vi "readSettingsFile.vi"(8 "error in (no error)":errorcluster, 10 "file (use dialog)":path, 11 "Controller in":refnum<class "Controller.lvclass">) -> (0 "error out":errorcluster, 3 "Controller out":refnum<class "Controller.lvclass">)   [LabVIEW 2019, in "Controller.lvclass"]
uses:
  Controller.lvclass
  Controller.lvclass/Controller.ctl
  Axis/Axis.lvclass
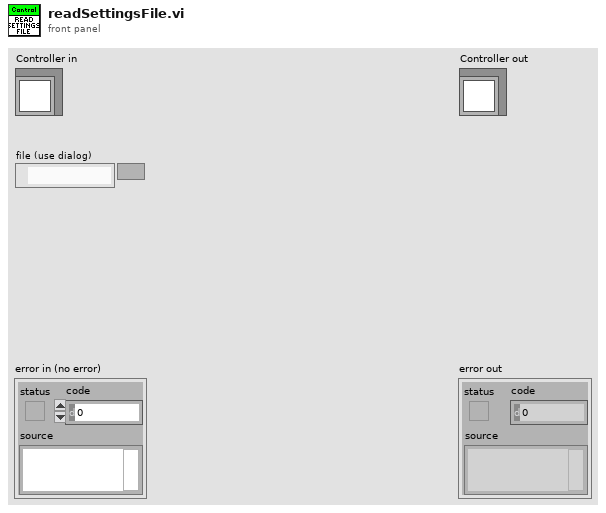
[diagram p1: front panel]
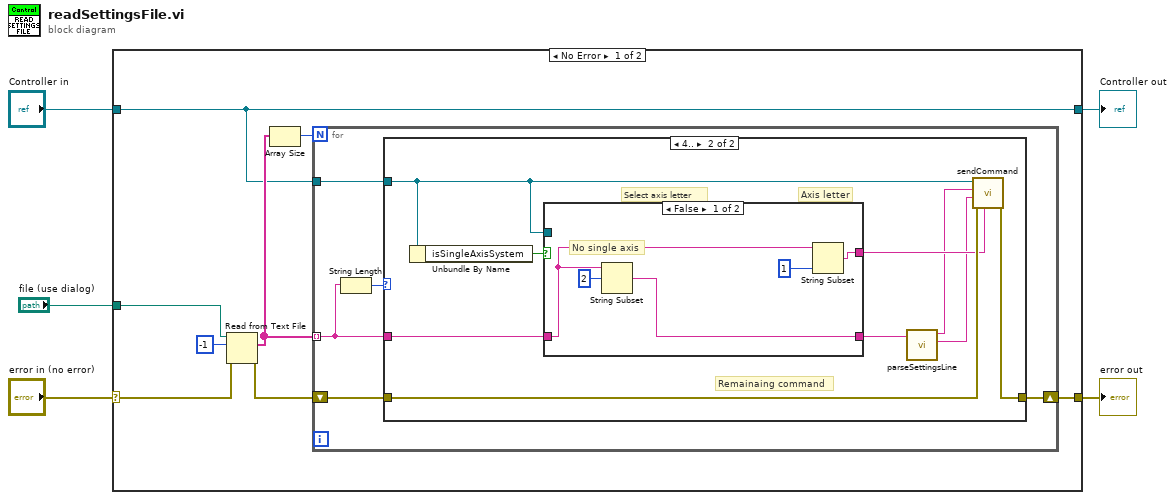
[diagram p0: block diagram]
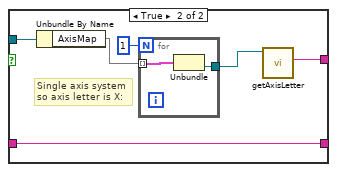
[diagram p3: hidden frame]
diagram:
  n1 = case shown="No Error" "error in (no error)" {
    selector: "error in (no error)" -> [w8 w43]
    tunnel: [w9 w43] -> w4
    tunnel: [w7 w42] -> w2
    tunnel: "Controller in" -> [w7 w42]
    tunnel: "file (use dialog)" -> [w6 _]
    frame No Error {
      n2 = Read from Text File(file (use dialog)=w6, count=-1, error in=w8) -> (text=w11:string[], error out=w10:errorcluster)  [unwired: 1 in, 2 out]
      n3 = Array Size(array=w11) -> (size(s)=w12:i32)
      n4 = for {
        N: w12 -> [_]
        tunnel: w11 -> [w17] mode=indexing
        shift-right: [w15] -> w9
        shift-left: w10 -> [w16]
        tunnel: w7 -> [w14]
        n5 = String Length(string=w17) -> (length=w18:i32)
        n6 = case shown="4.." w18 {
          tunnel: w17 -> [_ w27]
          tunnel: w16 -> [w19 w25]
          tunnel: [w19 w24] -> w15
          tunnel: w14 -> [_ w26]
          frame 0, Default {
          }
          frame 4.. {
            # "Remainaing command"
            # "Axis letter"
            # "Select axis letter"
            n7 = Unbundle By Name(w26) -> ("isSingleAxisSystem"=w28:bool)
            n8 = case shown="False" w28 {
              tunnel: w27 -> [w30 w39]
              tunnel: [w29 w39] -> w20
              tunnel: [w32 w37] -> w23
              tunnel: w26 -> [_ w38]
              frame False {
                # "No single axis"
                n9 = String Subset(string=w30, offset (0)=2) -> (substring=w29:string)  [unwired: 1 in]
                n10 = String Subset(string=w30, length (rest)=1) -> (substring=w32:string)  [unwired: 1 in]
              }
              frame True {
                # "Single axis system \nso axis letter is X:"
                n11 = Unbundle By Name(w38) -> ("AxisMap"=w34:map{string, refnum<class "Axis.lvclass">})
                n12 = for {
                  N: 1 -> [_]
                  tunnel: w34 -> [w41] mode=indexing
                  tunnel: [w40] -> w35
                  n13 = Unbundle(w41) -> ("Axis.lvclass"=w40:refnum<class "Axis.lvclass">)  [unwired: 1 out]
                }
                n14 = call-dynamic "getAxisLetter.vi"("Axis in"=w35) -> ("Axis Letter"=w37:string)  [unwired: 8 in, 2 out]
              }
            }
            n15 = call "parseSettingsLine.vi"("String"=w20) -> ("value"=w21:string, "key"=w22:string)  [unwired: 8 in, 1 out]
            n16 = call-dynamic "sendCommand.vi"("Axis Letter"=w23, "error in (no error)"=w25, "Value"=w21, "Command"=w22, "Controller in"=w26) -> ("error out"=w24:errorcluster)  [unwired: 5 in, 1 out]
          }
        }
      }
    }
    frame Error {
    }
  }
  "error out" <- w4
  "Controller out" <- w2
